vi "vision2.vi"(0 "Color Plane (Color Plane Extraction 1)":i32(ring)=2 items=["Red", "Green", "Blue", "Hue", "Saturation", "Luminance", "Value", "Intensity"], 1 "Range (Threshold 1)":cluster{"Lower value":sgl, "Upper value":sgl}={"Lower value"=199.0, "Upper value"=255.0}, 2 "Number of Erosion (Adv. Morphology 1)":i32=1, 3 "Square/Hexa (Square) (Adv. Morphology 1)":bool, 4 "Connectivity 4/8 (8) (Adv. Morphology 1)":bool=TRUE, 5 "Low Pass/High Pass (Low) (Adv. Morphology 1)":bool, 7 "error in":errorcluster) -> (20 "Centroid (Centroid 1)":cluster{"X Centroid":sgl, "Y Centroid":sgl} {"Y Centroid" format="%.2f"; "X Centroid" format="%.2f"}, 21 "Calibrated Centroid (Centroid 1)":cluster{"X Centroid":sgl, "Y Centroid":sgl} {"Y Centroid" format="%.2f"; "X Centroid" format="%.2f"}, 27 "error out":errorcluster)   [LabVIEW 2016]
uses:
  <vilib>/vision/driver/NI_Vision_Acquisition_Software.lvlib
  <vilib>/vision/NI_Vision_Development_Module.lvlib
panel:
  out "Image Out":T1(plugin-control)
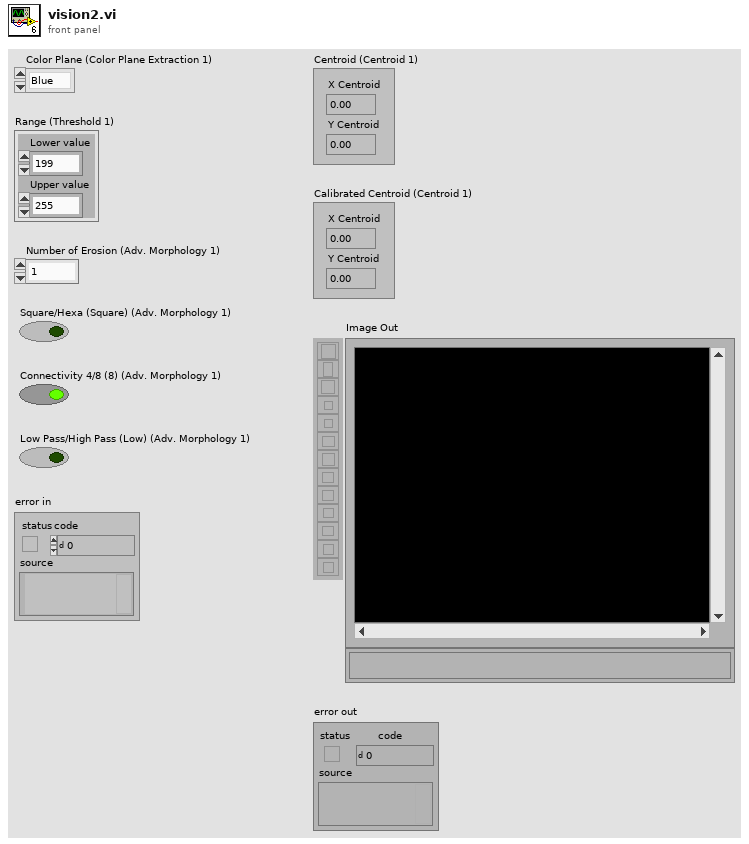
[diagram p1: front panel]
types:
  T1 = typedef "IMAQ Image.ctl" = refnum<image>
  T2 = typedef "IMAQdx.ctl" = refnum<k21>
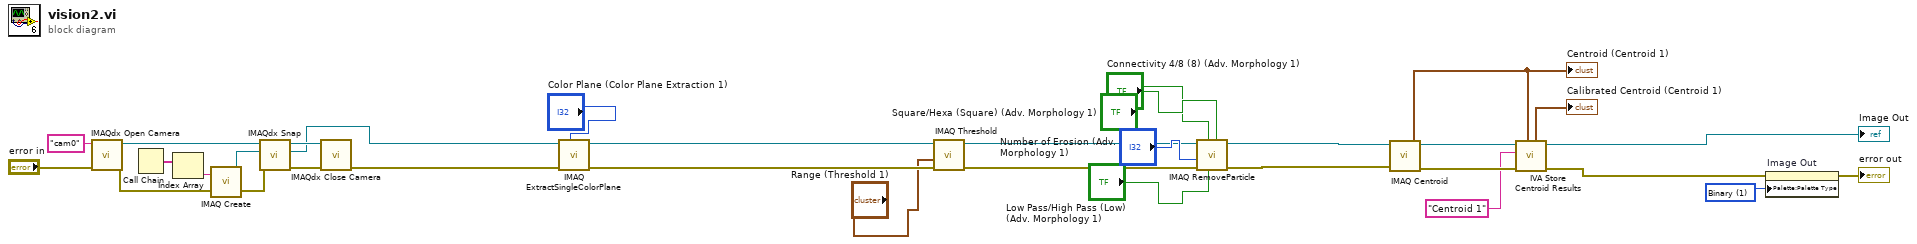
[diagram p0: block diagram]
diagram:
  w1 = u32 1 items=["Grayscale", "Binary", "Gradient", "Rainbow", "Temperature", "User Defined", "Binary 16 Bit", "Gradient 16 Bit", "Rainbow 16 Bit", "Temperature 16 Bit", "User Defined 16 Bit"] ("Palette Type")
  n1 = call <vilib>:"IMAQdx Open Camera.vi"("error in"="error in", "Session In"="cam0" ("Interface Name")) -> ("error out"=w31:errorcluster, "Session Out"=w25:T2)  [unwired: 1 in, 7 out]
  n2 = Call Chain() -> (call chain=w23:string[])
  n3 = Index Array(array=w23) -> (element=w22:string)  [unwired: 1 in]
  n4 = call "IMAQ Create"("Image Name"=w22, "error in (no error)"=w31) -> ("New Image"=w27:T1, "error out"=w26:errorcluster)  [unwired: 2 in, 1 out]
  n5 = call <vilib>:"IMAQdx Snap.vi"("error in"=w26, "Image In"=w27, "Session In"=w25) -> ("error out"=w29:errorcluster, "Image Out"=w20:T1, "Session Out"=w30:T2)  [unwired: 6 out]
  n6 = call <vilib>:"IMAQdx Close Camera.vi"("error in"=w29, "Session In"=w30) -> ("error out"=w28:errorcluster)  [unwired: 9 out]
  n7 = call "IMAQ ExtractSingleColorPlane"("Color Plane"="Color Plane (Color Plane Extraction 1)", "error in (no error)"=w28, "Image Src"=w20) -> ("error out"=w19:errorcluster, "Image Dst Out"=w17:T1)  [unwired: 1 in, 6 out]
  n8 = call "IMAQ Threshold"("error in (no error)"=w19, "Range"="Range (Threshold 1)", "Image Src"=w17) -> ("error out"=w16:errorcluster, "Image Dst Out"=w11:T1)  [unwired: 3 in, 4 out]
  n9 = call "IMAQ RemoveParticle"("Connectivity 4/8 (8)"="Connectivity 4/8 (8) (Adv. Morphology 1)", "Low Pass/High Pass (Low)"="Low Pass/High Pass (Low) (Adv. Morphology 1)", "Square/Hexa (Square)"="Square/Hexa (Square) (Adv. Morphology 1)", "error in (no error)"=w16, "Number of Erosion"="Number of Erosion (Adv. Morphology 1)", "Image Src"=w11) -> ("error out"=w10:errorcluster, "Image Dst Out"=w7:T1)  [unwired: 1 in, 3 out]
  n10 = call "IMAQ Centroid"("error in (no error)"=w10, "Image"=w7) -> ("error out"=w9:errorcluster, "Centroid"=w5:cluster{"X Centroid":sgl, "Y Centroid":sgl})  [unwired: 1 in, 1 out]
  "Centroid (Centroid 1)" <- w5
  n11 = call <vilib>:"IVA Store Centroid Results.vi"("Centroid in"=w5, "error in (no error)"=w9, "Step Name"="Centroid 1", "Image in"=w7) -> ("error out"=w8:errorcluster, "Image dup"=→"Image Out":T1, "Calibrated Centroid"=→"Calibrated Centroid (Centroid 1)":cluster{"X":sgl, "Y":sgl})  [unwired: 5 out]
  n12 = property on="Image Out" class="ImageControl"(error in=w8, "Palette:Palette Type"=w1) -> (error out=→"error out":errorcluster)  [unwired: 1 in, 1 out]
